vi "keithley binary data read.vi"() -> ()   [LabVIEW 2020, in "Keithley 24xx.lvclass"]
uses:
  Instruments/Power Supply/Keithley 24xx/Keithley 24xx.lvclass
panel:
  out "*(type *) &x":sgl
  out "substring 3":string
  out "substring 2":string
  out "substring":string
  out "length 2":i32
  out "length":i32
  in  "read buffer":string="#0ff6@°\bž,î\u001b•~ ü`É\u0000\b F\n"
  out "data string":string
  out "array type (2D Dbl) 2":sgl[](array[numeric])
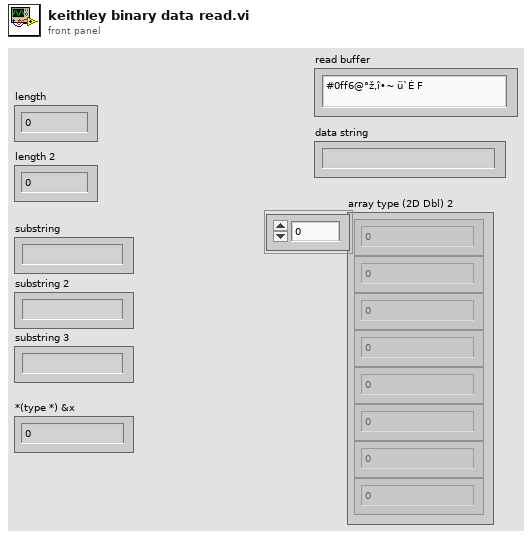
[diagram p1: front panel]
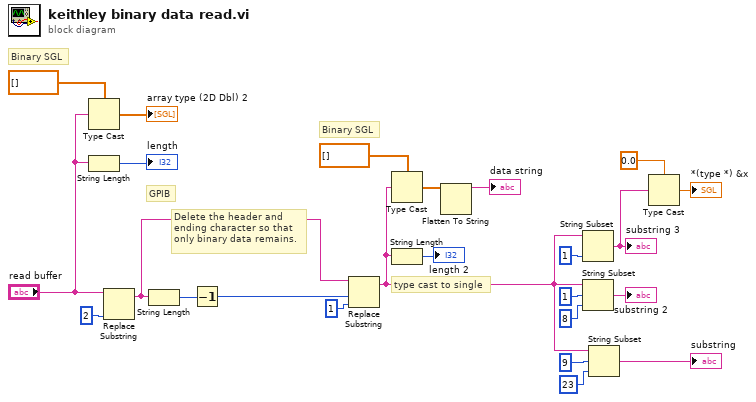
[diagram p0: block diagram]
diagram:
  # "Binary SGL"
  # "Delete the header and ending character so that only binary data remains."
  # "GPIB"
  # "type cast to single"
  # "Binary SGL"
  n1 = Type Cast(type=sgl[] [], x="read buffer") -> (*(type *) &x=→"array type (2D Dbl) 2":sgl[])
  n2 = String Length(string="read buffer") -> (length=→"length":i32)
  n3 = Replace Substring(2:2 ("length (len. of substring)"), 5:"read buffer") -> (1:w19:string)  [unwired: 2 in, 1 out]
  n4 = String Length(string=w19) -> (length=w18:i32)
  n5 = Decrement(x=w18) -> (x-1=w17:i32)
  n6 = Replace Substring(2:1 ("length (len. of substring)"), 3:w17, 5:w19) -> (1:w10:string)  [unwired: 1 in, 1 out]
  n7 = Type Cast(type=sgl[] [], x=w10) -> (*(type *) &x=w13:sgl[])
  n8 = String Length(string=w10) -> (length=→"length 2":i32)
  n9 = Flatten To String(anything=w13) -> (data string=→"data string":string)  [unwired: 3 in, 2 out]
  n10 = String Subset(string=w10, length (rest)=1 ("length (rest)")) -> (substring=w3:string)  [unwired: 1 in]
  "substring 3" <- w3
  n11 = String Subset(string=w10, offset (0)=1 ("length (rest)"), length (rest)=8 ("length (rest)")) -> (substring=→"substring 2":string)
  n12 = String Subset(string=w10, offset (0)=9 ("length (rest)"), length (rest)=23 ("length (rest)")) -> (substring=→"substring":string)
  n13 = Type Cast(type=sgl 0.0, x=w3) -> (*(type *) &x=→"*(type *) &x":sgl)
